vi "WFDC Get Correlation.vi"(0 "Center Ref Image":T1, 2 "Half Shift":i32=7, 7 "Current Image":u16[][](array[numeric]), 11 "Error In":errorcluster) -> (4 "Max Corr Value":dbl, 15 "Error Out":errorcluster)   [LabVIEW 2020]
uses:
  <vilib>/vision/Image Controls.llb/IMAQ Image.ctl
  WFDC DLL and Testing/Visual Studio NCC Max Shift DLL/x64/Release/VSmaxShiftNCC.dll
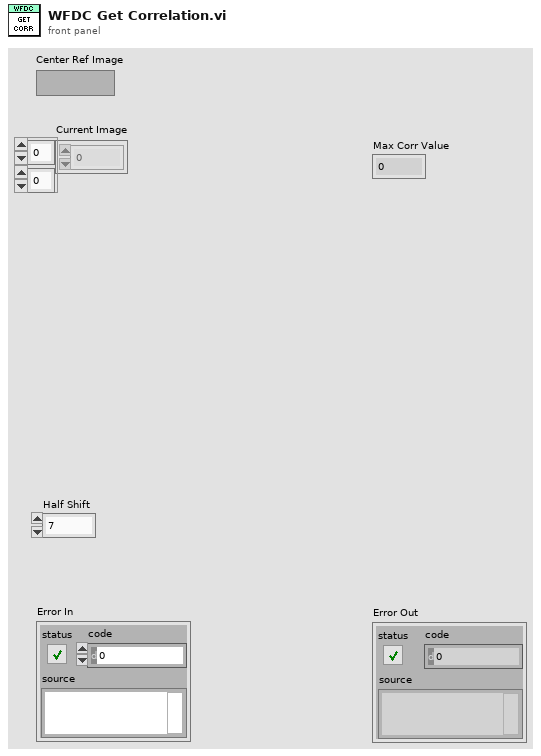
[diagram p1: front panel]
types:
  T1 = typedef "IMAQ Image.ctl" = refnum<image>
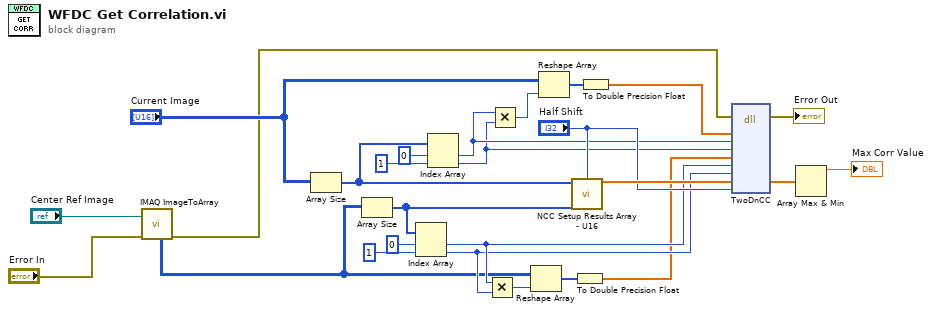
[diagram p0: block diagram]
diagram:
  n1 = call "IMAQ ImageToArray"("error in (no error)"="Error In", "Image"="Center Ref Image") -> ("Image Pixels (U16)"=w4:u16[][], "error out"=w24:errorcluster)  [unwired: 2 in, 3 out]
  n2 = Array Size(array="Current Image") -> (size(s)=w11:i32[])
  n3 = Array Size(array=w4) -> (size(s)=w5:i32[])
  n4 = Index Array(array=w5, index #1=0 ("index"), index #2=1 ("index")) -> (element #1=w18:i32, element #2=w17:i32)
  n5 = Index Array(array=w11, index #1=0 ("index"), index #2=1 ("index")) -> (element #1=w8:i32, element #2=w7:i32)
  n6 = Multiply(x=w18, y=w17) -> (x*y=w16:i32)
  n7 = Multiply(x=w8, y=w7) -> (x*y=w6:i32)
  n8 = Reshape Array(w4, w16) -> (w15:u16[])
  n9 = Reshape Array("Current Image", w6) -> (w10:u16[])
  n10 = call "NCC Setup Results Array - U16.vi"("Image 01 Size"=w11, "Half Shift"="Half Shift", "Image 02 Size"=w5) -> ("NCC Results Array"=w22:dbl[])  [unwired: 10 in, 2 out]
  n11 = To Double Precision Float(number=w15) -> (double precision float=w14:dbl[])
  n12 = To Double Precision Float(number=w10) -> (double precision float=w9:dbl[])
  n13 = dll-call lib="C:/Users/George Sirinakis/Documents/Microscope-Control/Microscope Modules/Wide Field Drift Correction/WFDC DLL and Testing/Visual Studio NCC Max Shift DLL/x64/Release/VSmaxShiftNCC.dll" fn="TwoDnCC"(error in=w24, "im01"=w9, "im01rowSize"=w8, "im01colSize"=w7, "im02"=w14, "im02rowSize"=w18, "im02ColSize"=w17, "theResult"=w22, "halfShift"="Half Shift") -> (error out=→"Error Out":errorcluster, "theResult"=w3:dbl[])  [unwired: 10 in, 1 out]
  n14 = Array Max & Min(array=w3) -> (max value=→"Max Corr Value":dbl)  [unwired: 3 out]
